vi "Voltmeter.vi"() -> ()   [LabVIEW 2023]
uses:
  PXIe-5172.lvclass
  Configurations/Voltmeter CFG/Voltmeter CFG/Voltmeter CFG.lvclass
  <userlib>/_OpenG.lib/file/file.llb/openg_file.lvlib
panel:
  out "filenames":string[](array[string])
  out "Error Out":errorcluster
  out "Waveform Chart":dbl(graph)
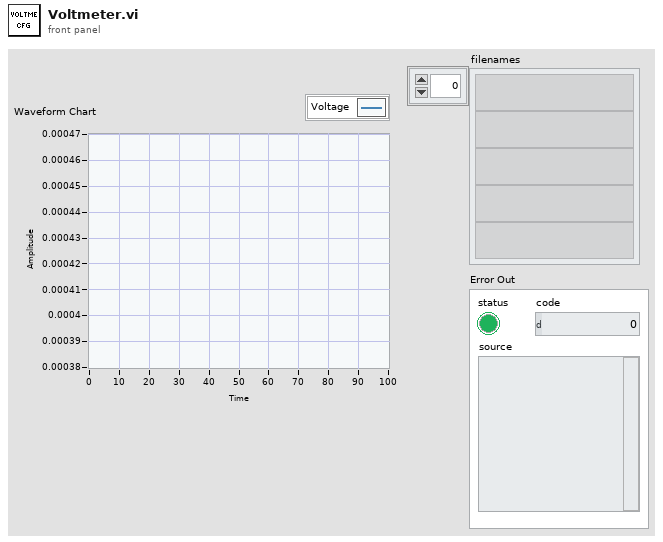
[diagram p1: front panel]
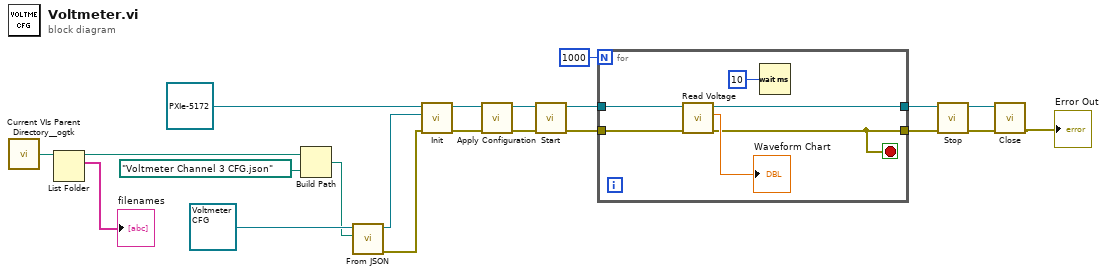
[diagram p0: block diagram]
diagram:
  n1 = call <userlib>:"Current VIs Parent Directory__ogtk.vi"() -> ("Parent Directory (+ Relative)"=w3:path)  [unwired: 5 in]
  n2 = List Folder(path=w3) -> (path out=w2:path, filenames=→"filenames":string[])  [unwired: 3 in, 2 out]
  n3 = Build Path(base path=w2, name or relative path=path "Voltmeter Channel 3 CFG.json") -> (appended path=w19:path)
  n4 = call-dynamic "From JSON.vi"("JSON Config"=w19, "object in"=refnum<class "Voltmeter CFG.lvclass"> refnum ("PXIe-5172.lvlib:Voltmeter CFG.lvclass")) -> ("error out"=w16:errorcluster, "object out"=w17:refnum<class "Voltmeter CFG.lvclass">)  [unwired: 8 in]
  n5 = call-dynamic "Init.vi"("Error In"=w16, "IConfigure"=w17, "object in"=refnum<class "PXIe-5172.lvclass"> refnum ("PXIe-5172.lvlib:PXIe-5172.lvclass")) -> ("Error Out"=w15:errorcluster, "object out"=w14:refnum<class "PXIe-5172.lvclass">)  [unwired: 7 in]
  n6 = call-dynamic "Apply Configuration.vi"("error in"=w15, "Scope Base in"=w14) -> ("error out"=w12:errorcluster, "Scope Base out"=w13:refnum<class "PXIe-5172.lvclass">)  [unwired: 8 in]
  n7 = call-dynamic "Start.vi"("error in"=w12, "Scope PXI in"=w13) -> ("error out"=w11:errorcluster, "Scope PXI out"=w10:refnum<class "PXIe-5172.lvclass">)  [unwired: 8 in]
  n8 = for {
    N: 1000 -> [_]
    tunnel: w11 -> [w27]
    tunnel: w10 -> [w26]
    tunnel: [w22] -> w8
    tunnel: [w24] -> w7
    stop <- w22 stop-if-true
    n9 = call-dynamic "Read Voltage.vi"("error in"=w27, "Scope Base in"=w26) -> ("error out"=w22:errorcluster, "Voltage"=→"Waveform Chart":dbl, "Scope Base out"=w24:refnum<class "PXIe-5172.lvclass">)  [unwired: 7 in]
    n10 = Wait (ms)(milliseconds to wait=u32 10) -> ()  [unwired: 1 out]
  }
  n11 = call-dynamic "Stop.vi"("error in (no error)"=w8, "Scope PXI in"=w7) -> ("error out"=w6:errorcluster, "Scope PXI out"=w5:refnum<class "PXIe-5172.lvclass">)  [unwired: 8 in]
  n12 = call-dynamic "Close.vi"("Error In"=w6, "object in"=w5) -> ("Error Out"=→"Error Out":errorcluster)  [unwired: 8 in, 1 out]
